vi "FTW-Inbox-Core-Callback.vi"(4 "Message Queue":T2 {"Routing Rules"."SendTimeout" format="%dmsec"; "Routing Rules"."BusyTimeout" format="%dmsec"}, 5 "Event Data":cluster{"Incoming Message Backtrace":i64} {"Incoming Message Backtrace" format="0x%016x"}, 6 "Incoming Message Event":refnum<user-event>, 7 "Common Event Data":T1) -> ()   [LabVIEW 2015]
uses:
  FTW-Inbox-Core-CallbackParameters.ctl
  json/core/FTW-JSON-Core-Structure.ctl
  FTW-Inbox-Core-RoutingRule.ctl
  json/FTW-JSON-UpdateMode.ctl
  error/FTW-ERR-ThrowError.vi
  error/FTW-ERR-CallChain.vi
  string/FTW-STR-ReplaceWhitespace.vi
  string/FTW-STR-Array-Delimit.vi
  regex/FTW-Regex-ReplaceAll.vi
panel:
  out "Messages Handled":i32
  # "Inputs"
  # "Debug"
  # "Outputs"
  # "This async callback\nhas no outputs"
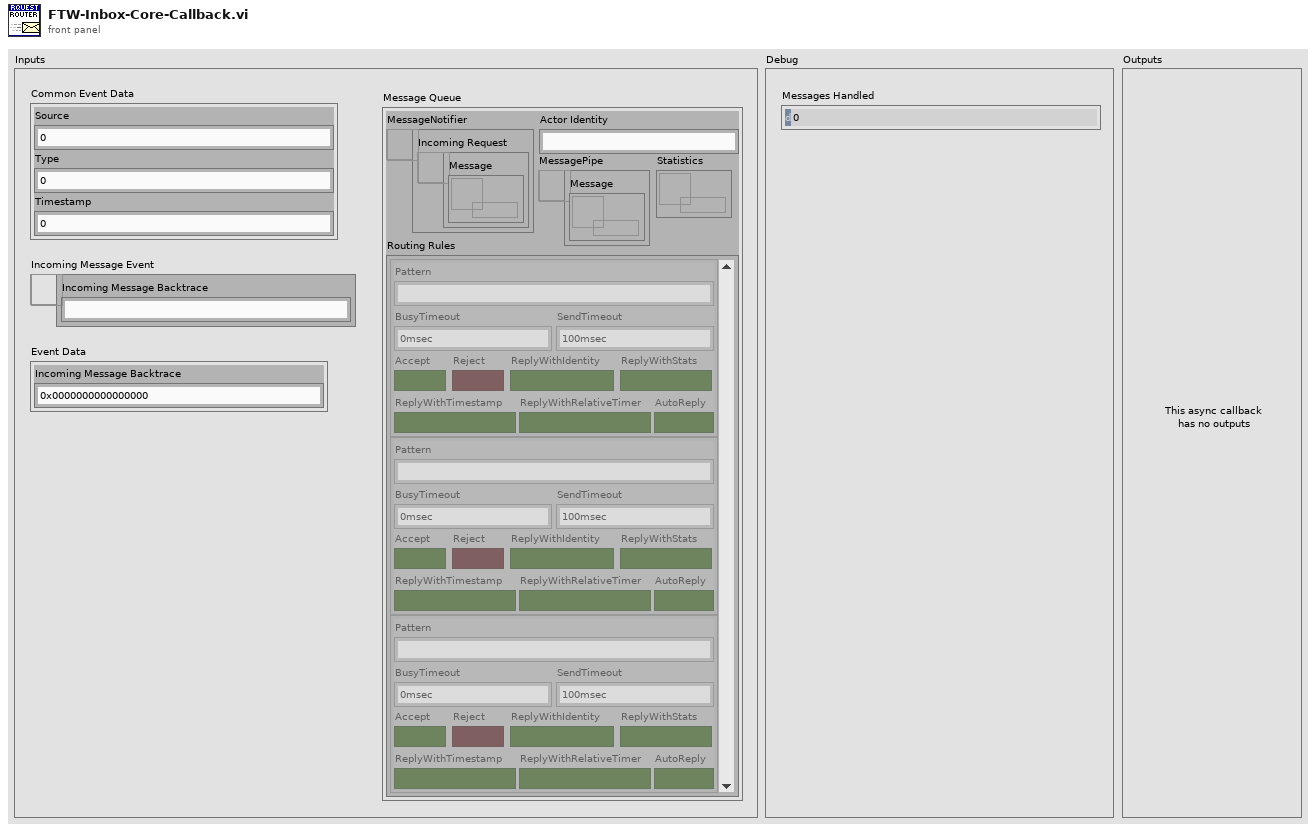
[diagram p1: front panel]
types:
  T1 = cluster{"Source":u32, "Type":u32, "Timestamp":u32}
  T2 = typedef "FTW-Inbox-Core-CallbackParameters.ctl" = cluster{"MessageNotifier":refnum<user-event>, "MessagePipe":refnum<queue>, "Routing Rules":T3[], "Actor Identity":string, "Statistics":refnum<data-value>}
  T3 = typedef "FTW-Inbox-Core-RoutingRule.ctl" = cluster{"Pattern":string, "BusyTimeout":i32, "SendTimeout":i32, "Accept":bool, "Reject":bool, "ReplyWithIdentity":bool, "ReplyWithStats":bool, "ReplyWithTimestamp":bool, "ReplyWithRelativeTimer":bool, "AutoReply":bool}
  T4 = typedef "FTW-JSON-Core-Structure.ctl" = cluster{"JSON Object":i64, "Encoding Flags":i64, "Decoding Flags":i64}
  T5 = cluster{"Backtrace":i64, "ReplyTimeout":i32, "ReponseIncludesTimestamp":bool, "ReponseIncludesRelativeTimer":bool, "ReponseIncludesException":bool}
  T6 = typedef "FTW-JSON-UpdateMode.ctl" = enum32{"Upsert", "Update Only", "Insert Only"}
  T7 = typedef "FTW-JSON-Type.ctl" = enum8{"Not Found", "Object", "Array", "String", "Number", "Boolean", "null"}
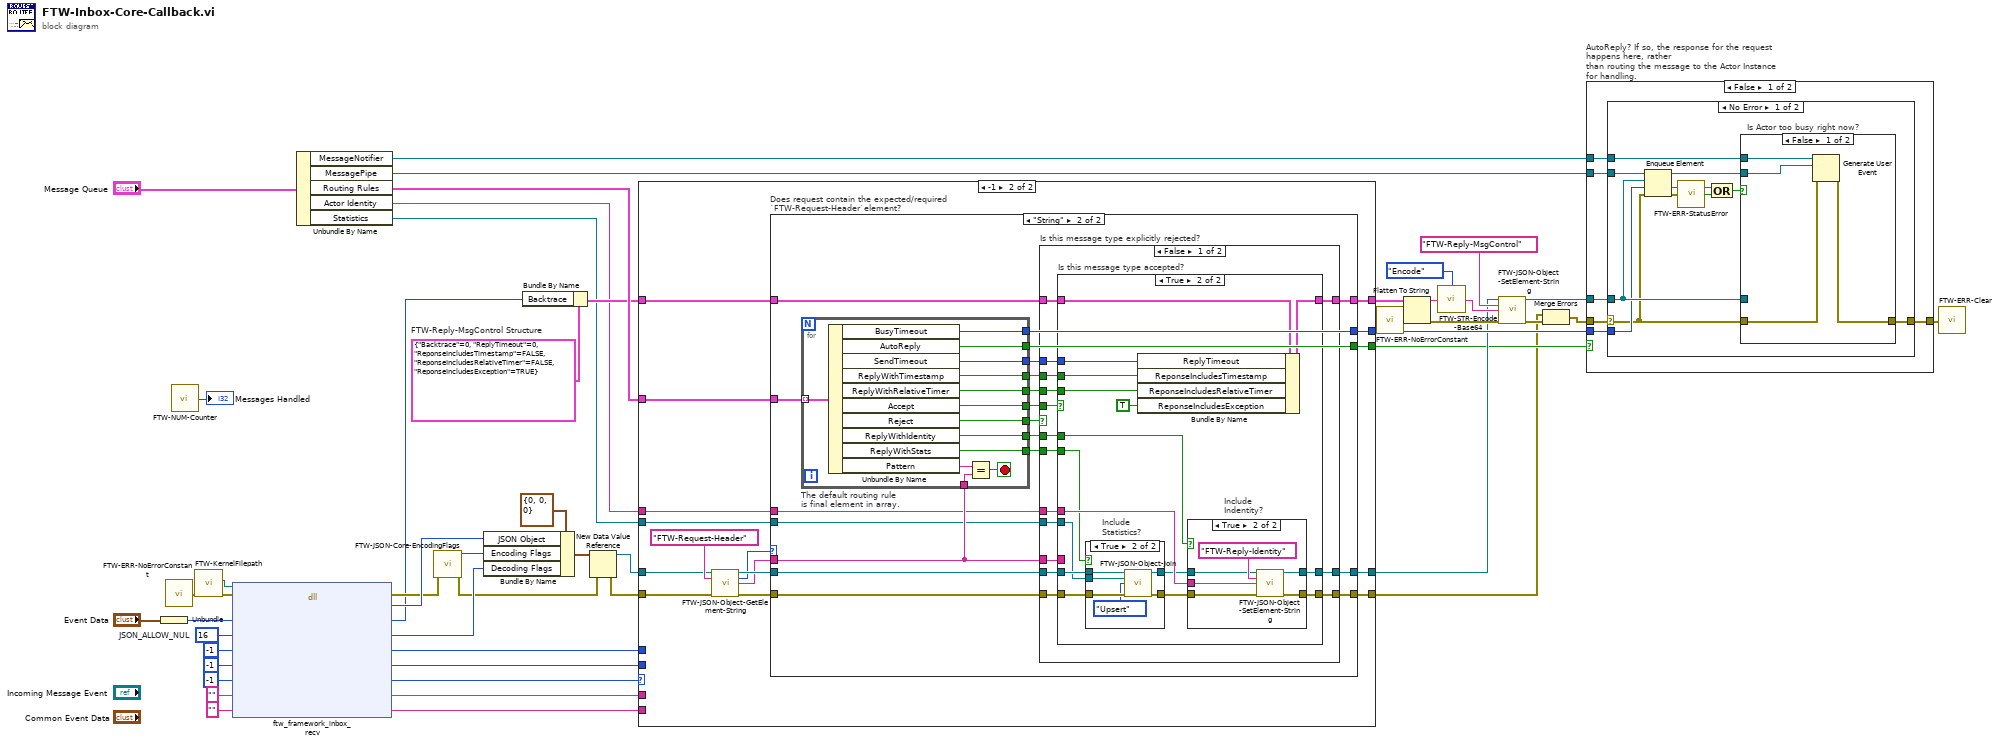
[diagram p0: block diagram]
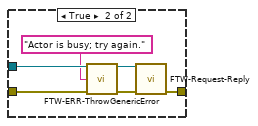
[diagram p2: hidden frame]
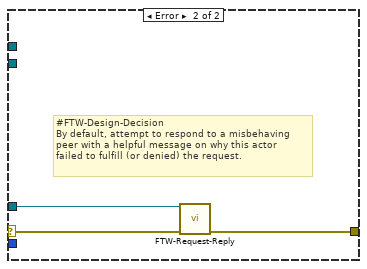
[diagram p3: hidden frame]
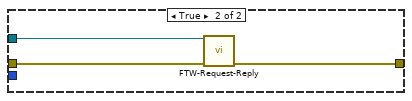
[diagram p4: hidden frame]
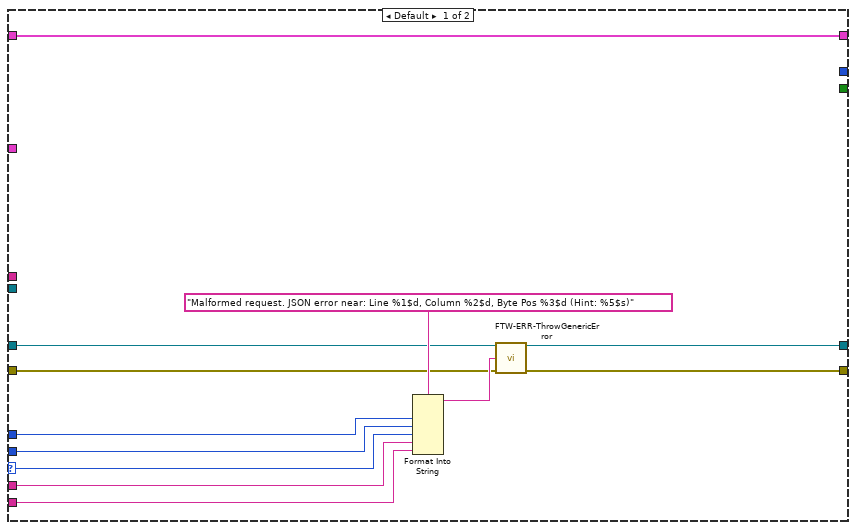
[diagram p5: hidden frame]
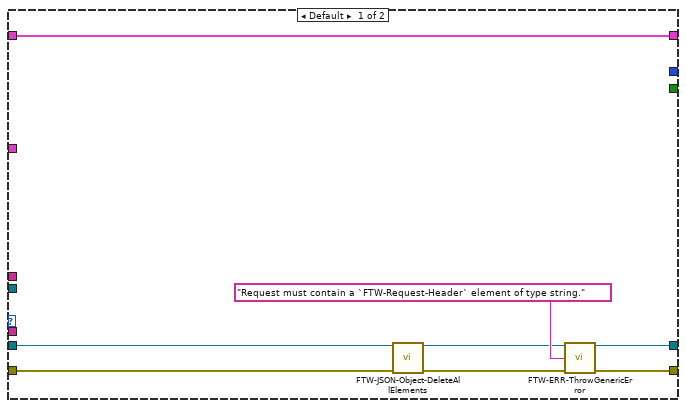
[diagram p6: hidden frame]
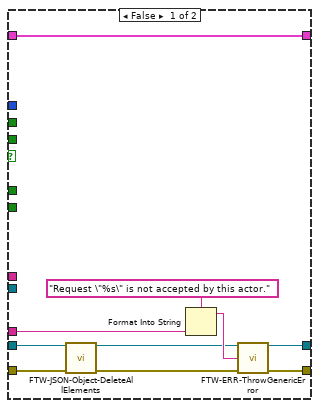
[diagram p7: hidden frame]
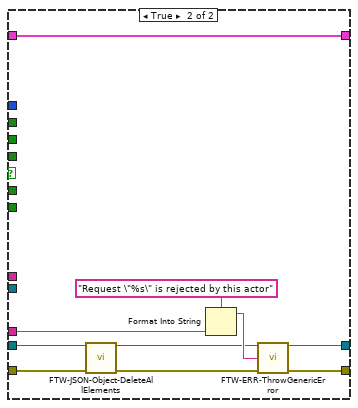
[diagram p10: hidden frame]
diagram:
  w23 = T5 {"Backtrace"=0, "ReplyTimeout"=0, "ReponseIncludesTimestamp"=FALSE, "ReponseIncludesRelativeTimer"=FALSE, "ReponseIncludesException"=TRUE}  # FTW-Reply-MsgControl Structure
  w38 = i64 16  # JSON_ALLOW_NUL
  n1 = Unbundle("Event Data") -> ("Incoming Message Backtrace"=w4:i64)
  n2 = call "FTW-ERR-NoErrorConstant.vi"() -> ("no error"=w3:errorcluster)
  n3 = call "FTW-NUM-Counter.vi"() -> ("Counter"=→"Messages Handled":i32)  [unwired: 1 in]
  n4 = call "FTW-KernelFilepath.vi"("error in"=w3) -> ("error out"=w2:errorcluster, "Library Filepath"=w1:path)  [unwired: 8 in, 1 out]
  n5 = dll-call lib="?" fn="ftw_framework_inbox_recv"(path in=w1, error in=w2, "Message Backtrace"=w4, "Flags"=w38, "Error Line Number"=i64 -1, "Error Column Number"=i64 -1, "Error Byte Position"=i64 -1, "Error Source"="", "Error Hint"="") -> (error out=w18:errorcluster, "JSON Object Pointer"=w19:i64, "Message Backtrace"=w12:i64, "Flags"=w17:i64, "Error Line Number"=w37:i64, "Error Column Number"=w36:i64, "Error Byte Position"=w13:i64, "Error Source"=w35:string, "Error Hint"=w34:string)  [unwired: 1 in, 1 out]
  n6 = Unbundle By Name("Message Queue") -> ("MessageNotifier"=w28:refnum<user-event>, "MessagePipe"=w29:refnum<queue>, "Routing Rules"=w33:T3[], "Actor Identity"=w11:string, "Statistics"=w10:refnum<data-value>)
  n7 = call "FTW-JSON-Core-EncodingFlags.vi"("error in"=w18) -> ("Encoding Flags"=w22:i64, "error out"=w16:errorcluster)  [unwired: 13 in]
  n8 = Bundle By Name(cluster=T4 {"JSON Object"=0, "Encoding Flags"=0, "Decoding Flags"=0}, "JSON Object"=w19, "Encoding Flags"=w22, "Decoding Flags"=w17) -> (w21:T4)
  n9 = Bundle By Name(cluster=w23, "Backtrace"=w12) -> (w32:T5)
  n10 = New Data Value Reference(data value=w21, error in=w16) -> (data value reference=w14:refnum<data-value>, error out=w15:errorcluster)
  n11 = case shown="-1" w13 {
    selector: w13 -> [w51 _]
    tunnel: [w53 w71] -> w6
    tunnel: w15 -> [w59 w66]
    tunnel: w37 -> [w58 _]
    tunnel: w36 -> [w57 _]
    tunnel: w35 -> [w56 _]
    tunnel: w34 -> [w55 _]
    tunnel: w33 -> [_ w74]
    tunnel: [w52 w72] -> w24
    tunnel: w32 -> [w54 w69]
    tunnel: [w54 w70] -> w31
    tunnel: [_ w68] -> w30
    tunnel: w11 -> [_ w67]
    tunnel: w14 -> [w52 w65]
    tunnel: w10 -> [_ w64]
    tunnel: [_ w62] -> w9
    frame Default {
      n12 = Format Into String(format string="Malformed request. JSON error near: Line %1$d, Column %2$d, Byte Pos %3$d (Hint: %5$s)", w58, w57, w51, w56, w55) -> (resulting string=w60:string)  [unwired: 2 in, 1 out]
      n13 = call "FTW-ERR-ThrowGenericError.vi"("Error Message"=w60, "error in"=w59) -> ("error out"=w53:errorcluster)  [unwired: 13 in]
    }
    frame -1 {
      n14 = call "FTW-JSON-Object-GetElement-String.vi"("JSON Object"=w65, "Key"="FTW-Request-Header", "error in"=w66) -> ("JSON Object out"=w75:refnum<data-value>, "JSON Element Type"=w63:T7, "Value"=w73:string, "error out"=w76:errorcluster)  [unwired: 9 in]
      n15 = case "Does request contain the expected/required `FTW-Request-Header`element?" shown="\"String\"" w63 {
        tunnel: w76 -> [w80 w103]
        tunnel: w75 -> [w82 w102]
        tunnel: [w81 w96] -> w72
        tunnel: [w83 w101] -> w71
        tunnel: w74 -> [_ w100]
        tunnel: w73 -> [_ w97]
        tunnel: [w78 w94] -> w70
        tunnel: w69 -> [w78 w95]
        tunnel: [_ w90] -> w68
        tunnel: w67 -> [_ w89]
        tunnel: w64 -> [_ w88]
        tunnel: [_ w85] -> w62
        frame Default {
          n16 = call "FTW-JSON-Object-DeleteAllElements.vi"("JSON Object"=w82, "error in"=w80) -> ("JSON Object out"=w81:refnum<data-value>, "error out"=w79:errorcluster)  [unwired: 12 in]
          n17 = call "FTW-ERR-ThrowGenericError.vi"("Error Message"="Request must contain a `FTW-Request-Header` element of type string.", "error in"=w79) -> ("error out"=w83:errorcluster)  [unwired: 13 in]
        }
        frame "String" {
          n18 = for "The default routing rule is final element in array." {
            tunnel: w100 -> [w181] mode=indexing
            tunnel: w97 -> [w179]
            tunnel: [w173] -> w99
            tunnel: [w174] -> w98
            tunnel: [w177] -> w93
            tunnel: [w176] -> w92
            tunnel: [w175] -> w91
            tunnel: [w170] -> w90
            tunnel: [w172] -> w87
            tunnel: [w171] -> w86
            tunnel: [w169] -> w85
            stop <- w178 stop-if-true
            n19 = Unbundle By Name(w181) -> ("BusyTimeout"=w170:i32, "AutoReply"=w169:bool, "SendTimeout"=w175:i32, "ReplyWithTimestamp"=w176:bool, "ReplyWithRelativeTimer"=w177:bool, "Accept"=w174:bool, "Reject"=w173:bool, "ReplyWithIdentity"=w172:bool, "ReplyWithStats"=w171:bool, "Pattern"=w180:string)
            n20 = Equal?(x=w180, y=w179) -> (x = y?=w178:bool)
          }
          n21 = case "Is this message type explicitly rejected?" shown="False" w99 {
            tunnel: w103 -> [w118 w163]
            tunnel: w102 -> [w117 w164]
            tunnel: [w116 w168] -> w101
            tunnel: w98 -> [w115 _]
            tunnel: w97 -> [w113 w165]
            tunnel: [w114 w161] -> w96
            tunnel: w95 -> [w112 w160]
            tunnel: [w111 w160] -> w94
            tunnel: w93 -> [w110 _]
            tunnel: w92 -> [w109 _]
            tunnel: w91 -> [w108 _]
            tunnel: w89 -> [w107 _]
            tunnel: w88 -> [w106 _]
            tunnel: w87 -> [w105 _]
            tunnel: w86 -> [w104 _]
            frame False {
              n22 = case "Is this message type accepted?" shown="True" w115 {
                tunnel: w118 -> [w124 w128]
                tunnel: w117 -> [w126 w133]
                tunnel: [w121 w136] -> w116
                tunnel: [w125 w137] -> w114
                tunnel: w113 -> [w120 _]
                tunnel: w112 -> [w119 w143]
                tunnel: [w119 w142] -> w111
                tunnel: w110 -> [_ w141]
                tunnel: w109 -> [_ w138]
                tunnel: w108 -> [_ w140]
                tunnel: w107 -> [_ w135]
                tunnel: w106 -> [_ w129]
                tunnel: w105 -> [_ w134]
                tunnel: w104 -> [_ w132]
                frame False {
                  n23 = call "FTW-JSON-Object-DeleteAllElements.vi"("JSON Object"=w126, "error in"=w124) -> ("JSON Object out"=w125:refnum<data-value>, "error out"=w122:errorcluster)  [unwired: 12 in]
                  n24 = Format Into String(format string="Request \"%s\" is not accepted by this actor." ("Error Message"), w120) -> (resulting string=w127:string)  [unwired: 2 in, 1 out]
                  n25 = call "FTW-ERR-ThrowGenericError.vi"("Error Message"=w127, "error in"=w122) -> ("error out"=w121:errorcluster)  [unwired: 13 in]
                }
                frame True {
                  n26 = case "Include\nStatistics?" shown="True" w132 {
                    tunnel: w133 -> [w145 w151]
                    tunnel: [w145 w150] -> w131
                    tunnel: [w144 w147] -> w130
                    tunnel: w128 -> [w144 w148]
                    tunnel: w129 -> [_ w149]
                    frame False {
                    }
                    frame True {
                      n27 = call "FTW-JSON-Object-Join.vi"("JSON Object"=w151, "JSON Object to Merge"=w149, "Join Mode"=FTW-JSON-UpdateMode."Upsert", "error in"=w148) -> ("JSON Object out"=w150:refnum<data-value>, "error out"=w147:errorcluster)  [unwired: 10 in]
                    }
                  }
                  n28 = Bundle By Name(cluster=w143, "ReplyTimeout"=w140, "ReponseIncludesTimestamp"=w138, "ReponseIncludesRelativeTimer"=w141, "ReponseIncludesException"=TRUE) -> (w142:T5)
                  n29 = case "Include\nIndentity?" shown="True" w134 {
                    tunnel: w131 -> [w153 w158]
                    tunnel: [w153 w157] -> w137
                    tunnel: [w152 w156] -> w136
                    tunnel: w130 -> [w152 w155]
                    tunnel: w135 -> [_ w154]
                    frame False {
                    }
                    frame True {
                      n30 = call "FTW-JSON-Object-SetElement-String.vi"("JSON Object"=w158, "Key"="FTW-Reply-Identity", "Value"=w154, "error in"=w155) -> ("JSON Object out"=w157:refnum<data-value>, "error out"=w156:errorcluster)  [unwired: 10 in]
                    }
                  }
                }
              }
            }
            frame True {
              n31 = call "FTW-JSON-Object-DeleteAllElements.vi"("JSON Object"=w164, "error in"=w163) -> ("JSON Object out"=w161:refnum<data-value>, "error out"=w162:errorcluster)  [unwired: 12 in]
              n32 = Format Into String(format string="Request \"%s\" is rejected by this actor" ("Error Message"), w165) -> (resulting string=w167:string)  [unwired: 2 in, 1 out]
              n33 = call "FTW-ERR-ThrowGenericError.vi"("Error Message"=w167, "error in"=w162) -> ("error out"=w168:errorcluster)  [unwired: 13 in]
            }
          }
        }
      }
    }
  }
  n34 = call "FTW-ERR-NoErrorConstant.vi"() -> ("no error"=w26:errorcluster)
  n35 = Flatten To String(anything=w31, error in (no error)=w26) -> (data string=w46:string, error out=w27:errorcluster)  [unwired: 2 in, 1 out]
  n36 = call "FTW-STR-Encode-Base64.vi"("Input"=w46, "Direction"=enum16{"Encode", "Decode"}."Encode") -> ("Output"=w44:string)
  n37 = call "FTW-JSON-Object-SetElement-String.vi"("JSON Object"=w24, "Key"="FTW-Reply-MsgControl", "Value"=w44, "error in"=w27) -> ("JSON Object out"=w8:refnum<data-value>, "error out"=w7:errorcluster)  [unwired: 10 in]
  n38 = Merge Errors(w6, w7) -> (w25:errorcluster)
  n39 = case "AutoReply? If so, the response for the request happens here, rather\nthan routing the message to the Actor Instance for handling." shown="False" w9 {
    tunnel: [w187 w211] -> w50
    tunnel: w30 -> [w186 _]
    tunnel: w29 -> [w185 _]
    tunnel: w28 -> [w184 _]
    tunnel: w25 -> [w183 w212]
    tunnel: w8 -> [w182 w213]
    frame False {
      n40 = case shown="No Error" w183 {
        selector: w183 -> [w188 w209]
        tunnel: w182 -> [w198 w210]
        tunnel: w186 -> [w197 _]
        tunnel: [w196 w208] -> w187
        tunnel: w185 -> [w191 _]
        tunnel: w184 -> [w190 _]
        frame No Error {
          n41 = Enqueue Element(queue=w191, element=w198, timeout in ms (-1)=w197, error in (no error)=w188) -> (queue out=w195:refnum<queue>, timed out?=w194:bool, error out=w192:errorcluster)
          n42 = call "FTW-ERR-StatusError.vi"("error to check"=w192) -> ("Error?"=w189:bool)
          n43 = Compound Arithmetic op=OR(w194, w189) -> (w193:bool)
          n44 = case "Is Actor too busy right now?" shown="False" w193 {
            tunnel: [w202 w207] -> w196
            tunnel: w190 -> [w201 _]
            tunnel: w188 -> [w200 w205]
            tunnel: w195 -> [w199 _]
            tunnel: w198 -> [_ w206]
            frame False {
              n45 = Generate User Event(user event=w201, event data cluster=w199, error in=w200) -> (error out=w202:errorcluster)  [unwired: 1 in, 1 out]
            }
            frame True {
              n46 = call "FTW-ERR-ThrowGenericError.vi"("Error Message"="Actor is busy; try again.", "error in"=w205) -> ("error out"=w204:errorcluster)  [unwired: 13 in]
              n47 = call "FTW-Request-Reply.vi"("Request"=w206, "error in"=w204) -> ("error out"=w207:errorcluster)  [unwired: 13 in]
            }
          }
        }
        frame Error {
          # "#FTW-Design-Decision\nBy default, attempt to respond to a misbehaving\npeer with a helpful message on why this actor\nfailed to fulfill (or denied) the request."
          n48 = call "FTW-Request-Reply.vi"("Request"=w210, "error in"=w209) -> ("error out"=w208:errorcluster)  [unwired: 13 in]
        }
      }
    }
    frame True {
      n49 = call "FTW-Request-Reply.vi"("Request"=w213, "error in"=w212) -> ("error out"=w211:errorcluster)  [unwired: 13 in]
    }
  }
  n50 = call "FTW-ERR-Clear.vi"("error to snuff"=w50) -> ()  [unwired: 1 out]
